vi "SequencerInitRS232.vi"(0 "VISA resource name":refnum<visa-resource-name>="COM7") -> (1 "error out":errorcluster, 2 "reference out":refnum<visa-resource-name>)   [LabVIEW 2014]
uses:
  <vilib>/Instr/_visa.llb/VISA Configure Serial Port (Instr).vi
panel:
  in  "XON Character":u8=17 format="%.0x"
  in  "XOFF Character":u8=19 format="%.0x"
  in  "Input\nbuffer size":u32=409600
  in  "flow control":u16(ring) items=["None"=0, "XON/XOFF"=1, "RTS/CTS"=2, "DTR/DSR"=4]
  in  "End write with termination character?":bool
  in  "termination char\n(0xA = '\\n' = LF)":u8=10 format="%.0x"
  in  "End read on termination character?":bool
  in  "timeout (ms)":u32=1000
  in  "stop bits":u16(ring)=20 items=["1.0"=10, "1.5"=15, "2.0"=20]
  in  "parity":u16(ring) items=["None", "Odd", "Even", "Mark", "Space"]
  in  "data bits":u16=8 min=5 max=8 step=1
  in  "baud rate":u32=4000000
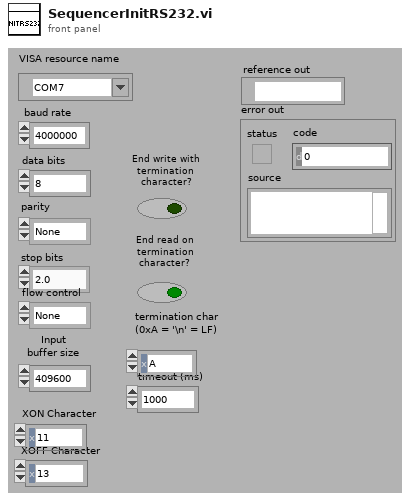
[diagram p1: front panel]
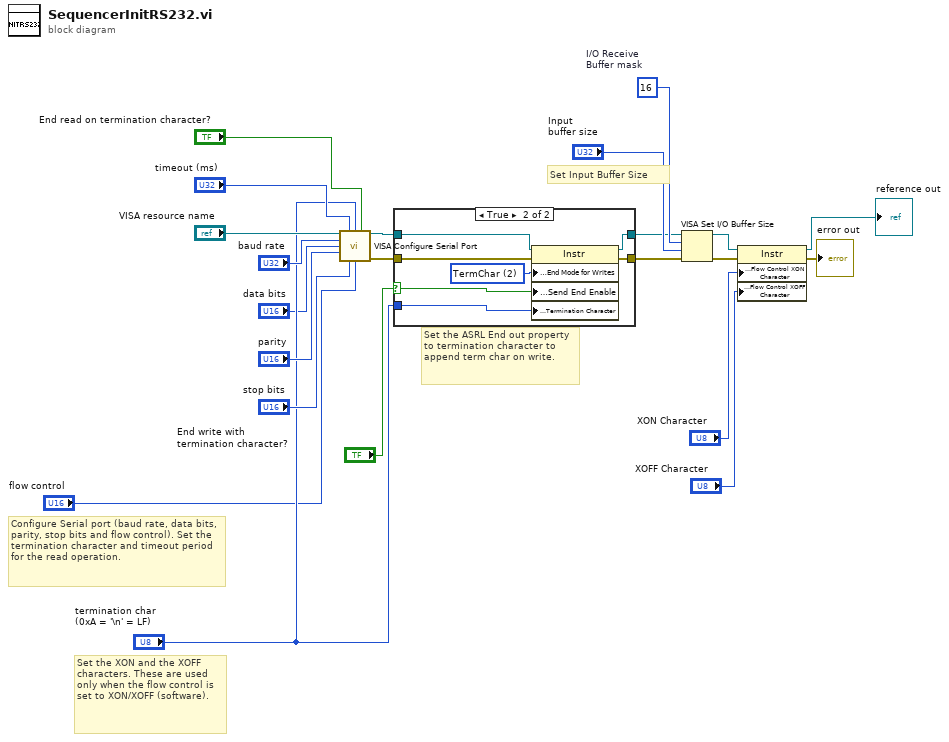
[diagram p0: block diagram]
diagram:
  w10 = u16 16  # I/O Receive Buffer mask
  # "Set the XON and the XOFF characters. These are used only when the flow control is set to XON/XOFF (software)."
  # "Set Input Buffer Size"
  # "Configure Serial port (baud rate, data bits, parity, stop bits and flow control). Set the termination character and timeout period for the read operation."
  # "Set the ASRL End out property to termination character to append term char on write."
  n1 = call-poly "VISA Configure Serial Port"("VISA resource name"="VISA resource name", "timeout (10sec)"="timeout (ms)", "termination char\n(0xA = '\\n' = LF)"="termination char\n(0xA = '\\n' = LF)", "Enable Termination\nChar (T)"="End read on termination character?", "baud rate (9600)"="baud rate", "data bits (8)"="data bits", "parity (0:none)"="parity", "stop bits (10: 1 bit)"="stop bits", "flow control (0:none)"="flow control") -> ("VISA resource name out"=w11:refnum<visa-resource-name>, "error out"=w12:errorcluster)  [unwired: 1 in, 4 out]
  n2 = case shown="True" "End write with termination character?" {
    selector: "End write with termination character?" -> [_ w25]
    tunnel: w11 -> [w23 w31]
    tunnel: w12 -> [w24 w30]
    tunnel: [w23 w29] -> w4
    tunnel: [w24 w28] -> w3
    tunnel: "termination char\n(0xA = '\\n' = LF)" -> [_ w26]
    frame False {
    }
    frame True {
      w27 = u16 2 items=["None", "LastBit", "TermChar", "Break"] ("Serial Settings:Serial End Mode for Writes")
      n3 = property class="Instr"(reference=w31, error in=w30, "Serial Settings:End Mode for Writes"=w27, "Message Based Settings:Send End Enable"=w25, "Message Based Settings:Termination Character"=w26) -> (reference out=w29:refnum<visa-resource-name>, error out=w28:errorcluster)
    }
  }
  n4 = VISA Set I/O Buffer Size(VISA resource name=w4, mask (16)=w10, size (4096)="Input\nbuffer size", error in (no error)=w3) -> (VISA resource name out=w8:refnum<visa-resource-name>, error out=w7:errorcluster)
  n5 = property class="Instr"(reference=w8, error in=w7, "Serial Settings:Flow Control XON Character"="XON Character", "Serial Settings:Flow Control XOFF Character"="XOFF Character") -> (reference out=→"reference out":refnum<visa-resource-name>, error out=→"error out":errorcluster)
